vi "Tools_String Close Calling VI's Windows.vi"(4 "error in (no error)":errorcluster, 6 "level (1)":i32=1, 7 "close (T)":bool) -> (0 "error out":errorcluster)   [LabVIEW 2017]
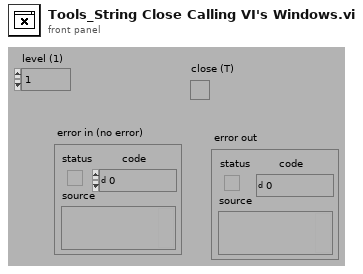
[diagram p1: front panel]
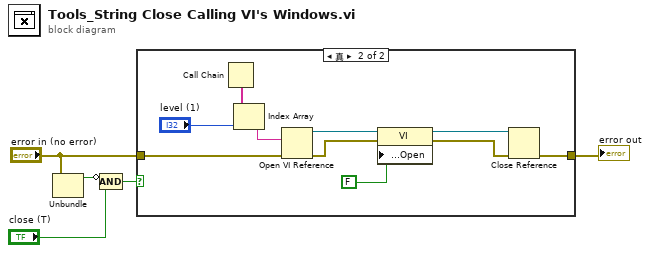
[diagram p0: block diagram]
diagram:
  n1 = Unbundle("error in (no error)") -> ("status"=w5:bool)  [unwired: 2 out]
  n2 = Compound Arithmetic op=AND(invert w5, "close (T)") -> (w2:bool)
  n3 = case shown="真" w2 {
    tunnel: "error in (no error)" -> [w6 w8]
    tunnel: [w6 w7] -> w1
    frame False {
    }
    frame True {
      n4 = Call Chain() -> (call chain=w16:string[])
      n5 = Index Array(array=w16, index="level (1)") -> (element=w9:string)
      n6 = Open VI Reference(vi path=w9, error in (no error)=w8) -> (vi reference=w14:refnum<vi>, error out=w11:errorcluster)  [unwired: 4 out]
      n7 = property class="VI"(reference=w14, error in=w11, "Front Panel Window:Open"=FALSE ("Front Panel.Open")) -> (reference out=w12:refnum<vi>, error out=w10:errorcluster)
      n8 = Close Reference(reference=w12, error in (no error)=w10) -> (error out=w7:errorcluster)
    }
  }
  "error out" <- w1
